vi "test_ao-1chNpt.vi"() -> ()   [LabVIEW 2019]
uses:
  _ctrl/cDAQ-9269 Config.ctl
  _ctrl/init-w-close.ctl
  _ctrl/rw.ctl
panel:
  out "error out":errorcluster
  in  "config":T1={"Ch"="Dev2/ao0", "Max V"=5.0, "Min V"=-5.0, " Rate"=1000.0, "N pts"=100, "sample mode"=2} {"sample mode" items=["유한 샘플"=10178, "연속 샘플"=10123, "하드웨어 타이밍에 의한 단일 포인트"=12522]}
  in  "AO signal":T2={"offset"=1.0, "signal type"=enum."Square Wave", "frequency"=10.0, "amplitude"=1.0, " duty"=50.0} {"amplitude" format="%0.2p"; "frequency" format="%.0p"; "offset" format="%0.2p"}
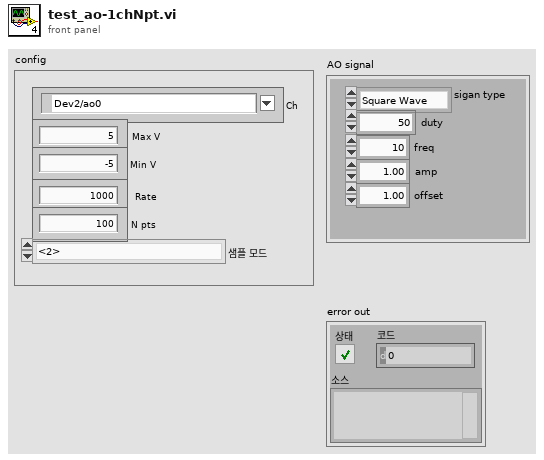
[diagram p1: front panel]
types:
  T1 = typedef "cDAQ-9269 Config.ctl" = cluster{"Ch":tag, "Max V":dbl, "Min V":dbl, " Rate":dbl, "N pts":i32, "sample mode":i32}
  T2 = cluster{"offset":dbl, "signal type":enum16{"Sine Wave", "Triangle Wave", "Square Wave", "Sawtooth Wave"}, "frequency":dbl, "amplitude":dbl, " duty":dbl}
  T3 = typedef "init-w-close.ctl" = enum16{"init", "write", "close"}
  T4 = typedef "rw.ctl" = enum16{"read", "write"}
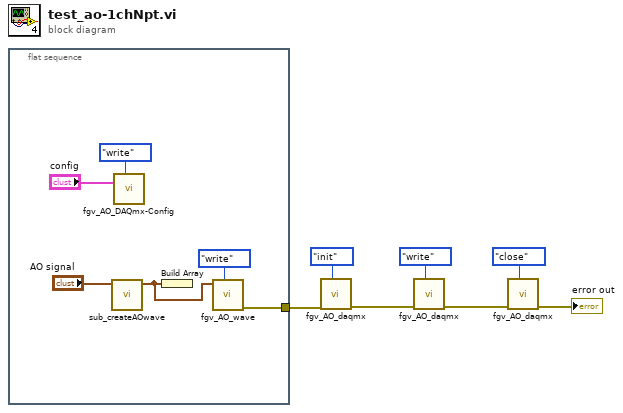
[diagram p0: block diagram]
diagram:
  n1 = flat-sequence {
    tunnel: [w11] -> w2
    frame #0 {
      n2 = call "sub_createAOwave.vi"("AO signal"="AO signal") -> ("AO wave"=w8:waveform(dbl))  [unwired: 10 in]
      n3 = call "fgv_AO_DAQmx-Config.vi"("cmd"=rw."write", "9269 AO Config"="config") -> ()  [unwired: 8 in, 2 out]
      n4 = Build Array(w8) -> ()  [unwired: 1 out]
      n5 = call "fgv_AO_wave.vi"("cmd"=rw."write", "signal in"=w8) -> ("error out"=w11:errorcluster)  [unwired: 8 in, 1 out]
    }
  }
  n6 = call "fgv_AO_daqmx.vi"("cmd"=init-w-close."init", "error in"=w2) -> ("error out"=w4:errorcluster)  [unwired: 9 in]
  n7 = call "fgv_AO_daqmx.vi"("cmd"=init-w-close."write", "error in"=w4) -> ("error out"=w3:errorcluster)  [unwired: 9 in]
  n8 = call "fgv_AO_daqmx.vi"("cmd"=init-w-close."close", "error in"=w3) -> ("error out"=→"error out":errorcluster)  [unwired: 9 in]
